vi "Create Section.vi"(7 "Section name":string, 8 "error in (no error)":errorcluster, 10 "Create section? [T]":bool=TRUE, 11 "Carya Config in":refnum<class "Carya Config.lvclass">) -> (0 "error out":errorcluster, 1 "Session excist?":bool, 2 "Created session?":bool, 3 "Carya Config out":refnum<class "Carya Config.lvclass">)   [LabVIEW 2013, in "Carya Config.lvclass"]
doc: "Copyright 2018, Carya Automatisering, Wiebe Walstra."
uses:
  Carya Config.lvclass
  CConfig Object/CConfig Query.lvclass
  CConfig Object/Loop Query/Match Query/Match Query.lvclass
  CConfig Object/Composite Query/Composite Query.lvclass
  CConfig Object/Add Results Query/Add Results Query.lvclass
  CConfig Object/Insert Query/Insert Query.lvclass
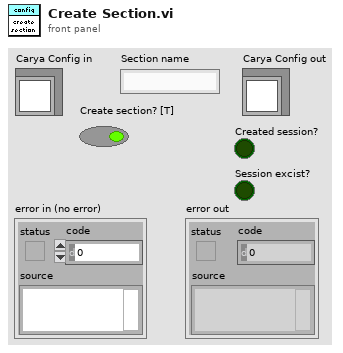
[diagram p1: front panel]
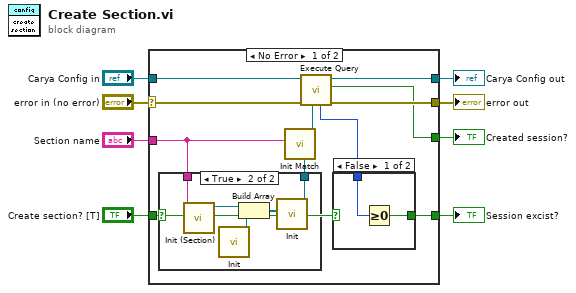
[diagram p0: block diagram]
diagram:
  n1 = case shown="No Error" "error in (no error)" {
    selector: "error in (no error)" -> [w19 w29]
    tunnel: [w18 w29] -> w7
    tunnel: [w16 w28] -> w5
    tunnel: "Carya Config in" -> [w17 w28]
    tunnel: "Section name" -> [w13 _]
    tunnel: "Create section? [T]" -> [w9 _]
    tunnel: [w12 _] -> w2
    tunnel: [w11 _] -> w1
    frame No Error {
      n2 = case shown="True" w9 {
        tunnel: [_ w27] -> w14
        tunnel: w13 -> [_ w23]
        frame False {
        }
        frame True {
          n3 = call "Init (Section).vi"("Name"=w23) -> ("Find First Query out"=w24:refnum<class "Insert Query.lvclass">)  [unwired: 9 in, 1 out]
          n4 = call "Init.vi"() -> ("Find First Query out"=w25:refnum<class "Add Results Query.lvclass">)  [unwired: 10 in, 1 out]
          n5 = Build Array(w24, w25) -> (w26:refnum<class "CConfig Query.lvclass">[])
          n6 = call "Init.vi"("Queries"=w26) -> ("Step In Query out"=w27:refnum<class "CConfig Query.lvclass">)  [unwired: 9 in, 1 out]
        }
      }
      n7 = call "Init Match.vi"("Not found"=w14, "Data"=w13) -> ("Find First Query out"=w15:refnum<class "Loop Query.lvclass">)  [unwired: 8 in, 1 out]
      n8 = call-dynamic "Execute Query.vi"("Config Query in"=w15, "error in (no error)"=w19, "Carya Config in"=w17) -> ("error out"=w18:errorcluster, "Result"=w12:bool, "Carya Config out"=w16:refnum<class "Carya Config.lvclass">, "Index"=w10:i32)  [unwired: 4 in, 1 out]
      n9 = case shown="False" w9 {
        selector: w9 -> [_ w22]
        tunnel: [w20 w22] -> w11
        tunnel: w10 -> [w21 _]
        frame False {
          n10 = Greater Or Equal To 0?(x=w21) -> (x >= 0?=w20:bool)
        }
        frame True {
        }
      }
    }
    frame Error {
    }
  }
  "error out" <- w7
  "Carya Config out" <- w5
  "Created session?" <- w2
  "Session excist?" <- w1
